vi "Merge Configuration.vi"(8 "error in (no error)":errorcluster, 10 "Additional Configuration":string, 11 "IO Class in":refnum<class "Signal.lvclass">) -> (0 "error out":errorcluster, 3 "IO Class out":refnum<class "Signal.lvclass">)   [LabVIEW 2015, in "Signal.lvclass"]
uses:
  Signal.lvclass
  Signal.lvclass/Signal.ctl
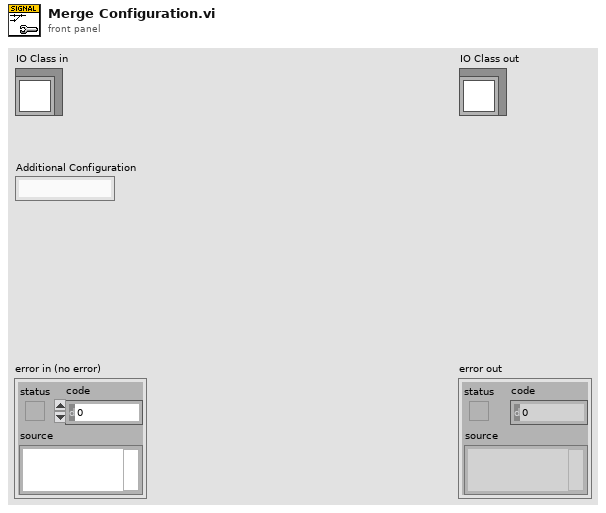
[diagram p1: front panel]
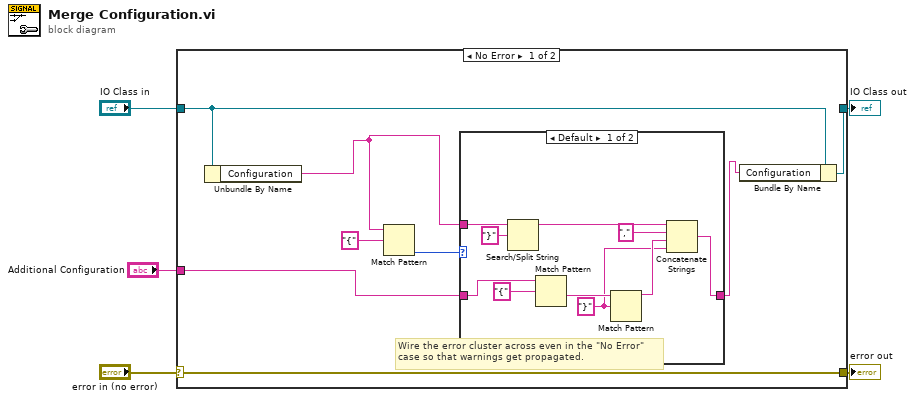
[diagram p0: block diagram]
diagram:
  n1 = case shown="No Error" "error in (no error)" {
    selector: "error in (no error)" -> [w13 w26]
    tunnel: [w13 w26] -> w4
    tunnel: [w7 w25] -> w2
    tunnel: "IO Class in" -> [w8 w25]
    tunnel: "Additional Configuration" -> [w6 _]
    frame No Error {
      # "Wire the error cluster across even in the \"No Error\"\ncase so that warnings get propagated."
      n2 = Unbundle By Name(w8) -> ("Configuration"=w10:string)
      n3 = Match Pattern(string=w10, regular expression="{") -> (offset past match=w11:i32)  [unwired: 1 in, 3 out]
      n4 = case shown="Default" w11 {
        tunnel: [w14 w24] -> w9
        tunnel: w6 -> [w20 w24]
        tunnel: w10 -> [w22 _]
        frame Default {
          w15 = "}" ("regular expression")
          n5 = Search/Split String(string=w22, search string/char (-)="}" ("regular expression")) -> (substring before match=w18:string)  [unwired: 1 in, 2 out]
          n6 = Match Pattern(string=w20, regular expression="{") -> (after substring=w19:string)  [unwired: 1 in, 3 out]
          n7 = Match Pattern(string=w19, regular expression=w15) -> (before substring=w16:string)  [unwired: 1 in, 3 out]
          n8 = Concatenate Strings(w18, "," ("string"), w16, w15) -> (w14:string)
        }
        frame -1 {
        }
      }
      n9 = Bundle By Name(cluster=w8, "Configuration"=w9) -> (w7:refnum<class "Signal.lvclass">)
    }
    frame Error {
    }
  }
  "error out" <- w4
  "IO Class out" <- w2
